vi "DeFUSeUploader.vi"(8 "Error In":errorcluster, 10 "DFU-Util Working Directory":path=path "", 11 "Binary Filename":path=path "") -> (0 "Error Out":errorcluster)   [LabVIEW 2010]
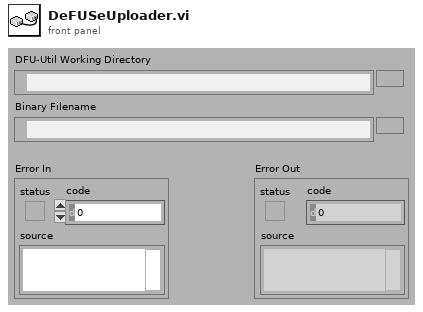
[diagram p1: front panel]
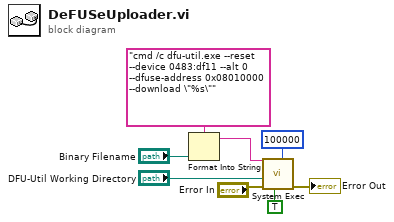
[diagram p0: block diagram]
diagram:
  n1 = Format Into String(format string="cmd /c dfu-util.exe --reset --device 0483:df11 --alt 0 --dfuse-address 0x08010000 --download \"%s\"", "Binary Filename") -> (resulting string=w4:string)  [unwired: 2 in, 1 out]
  n2 = call <vilib>:"System Exec.vi"("expected output size  (4096)"=u32 100000, "run minimized? (F)"=TRUE, "error in (no error)"="Error In", "working directory"="DFU-Util Working Directory", "command line"=w4) -> ("error out"=→"Error Out":errorcluster)  [unwired: 3 in, 3 out]
